vi "zad1.vi"() -> ()   [LabVIEW 2017]
panel:
  out "String":string
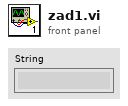
[diagram p1: front panel]
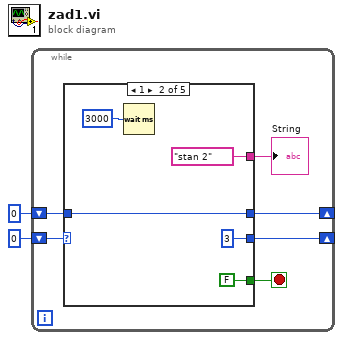
[diagram p0: block diagram]
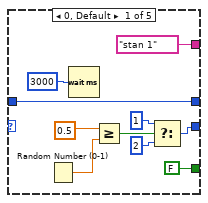
[diagram p2: hidden frame]
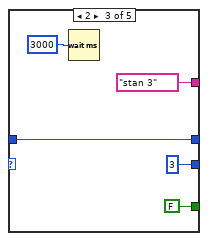
[diagram p3: hidden frame]
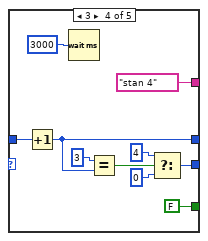
[diagram p4: hidden frame]
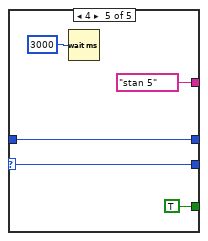
[diagram p5: hidden frame]
diagram:
  n1 = while {
    shift-right: [w6] -> _
    shift-left: 0 -> [w7]
    shift-right: [w4] -> _
    shift-left: 0 -> [w5]
    stop <- w3 stop-if-true
    n2 = case shown="1" w7 {
      selector: w7 -> [_ _ _ _ w41]
      tunnel: ["stan 1" "stan 2" "stan 3" "stan 4" "stan 5"] -> w8
      tunnel: [w13 3 3 w31 w41] -> w6
      tunnel: w5 -> [w12 w20 w25 w36 w40]
      tunnel: [w12 w20 w25 w30 w40] -> w4
      tunnel: [FALSE FALSE FALSE FALSE TRUE] -> w3
      frame 0, Default {
        n3 = Random Number (0-1)() -> (number: 0 to 1=w9:dbl)
        n4 = Wait (ms)(milliseconds to wait=3000) -> ()  [unwired: 1 out]
        n5 = Greater Or Equal?(x=0.5, y=w9) -> (x >= y?=w16:bool)
        n6 = Select(t=1, s=w16, f=2) -> (s? t:f=w13:i32)
      }
      frame 1 {
        n7 = Wait (ms)(milliseconds to wait=3000) -> ()  [unwired: 1 out]
      }
      frame 2 {
        n8 = Wait (ms)(milliseconds to wait=3000) -> ()  [unwired: 1 out]
      }
      frame 3 {
        n9 = Increment(x=w36) -> (x+1=w30:i32)
        n10 = Wait (ms)(milliseconds to wait=3000) -> ()  [unwired: 1 out]
        n11 = Equal?(x=3, y=w30) -> (x = y?=w34:bool)
        n12 = Select(t=4, s=w34, f=0) -> (s? t:f=w31:i32)
      }
      frame 4 {
        n13 = Wait (ms)(milliseconds to wait=3000) -> ()  [unwired: 1 out]
      }
    }
    "String" <- w8
  }
